vi "DzMod_ErrorCodes&Descs.vi"() -> (0 "AV_ErrorsDescs_Trans":cluster{"Code":i32, "Description":string}[](array[cluster])=[{"Code"=25001, "Description"="Waveform would be truncated in time domain by the Dazzler."}, {"Code"=25002, "Description"="Waveform amplitude would exceed the maximum acceptable by RF generator."}] caption="Error Descriptions")   [LabVIEW 2012]
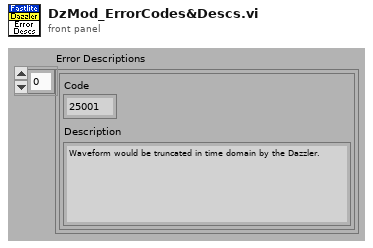
[diagram p1: front panel]
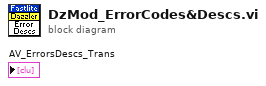
[diagram p0: block diagram]
diagram:
